vi "Quick Usb Write RS232.vi"(7 "length":u16, 8 "error in (no error)":errorcluster, 9 "data":string, 10 "portNum":u8, 11 "hDevice":u32) -> (0 "error out":errorcluster, 1 "data out":string, 2 "function return":i32, 3 "hDevice out":u32)   [LabVIEW 2011, in "QuickUSB.lvlib"]
doc: "QUSBLIB QRETURN QuickUsbWriteRS232(\n QHANDLE hDevice, \n QBYTE portNum, \n PQBYTE data, \n QWORD length\n);"
uses:
  QuickUSB.lvlib
  QuickUSB.dll
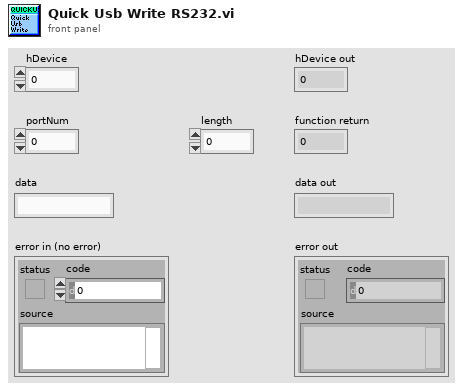
[diagram p1: front panel]
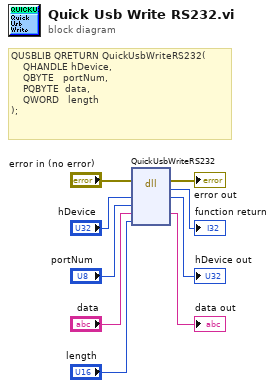
[diagram p0: block diagram]
diagram:
  # "QUSBLIB QRETURN QuickUsbWriteRS232(\n    QHANDLE hDevice, \n    QBYTE   portNum, \n    PQBYTE  data, \n    QWORD   length\n);"
  n1 = dll-call lib="C:/QuickUSB/QuickUSB.*" fn="QuickUsbWriteRS232"(error in="error in (no error)", "hDevice"="hDevice", "portNum"="portNum", "data"="data", "length"="length") -> (error out=→"error out":errorcluster, →"function return":i32, "hDevice"=→"hDevice out":u32, "data"=→"data out":string)  [unwired: 4 in, 1 out]
